vi "喷码内容转换.vi"(10 "输入数据(十进制)":string="123456789") -> (2 "输出数据(十六进制)":string)   [LabVIEW 2020, in "Untitled Library 1.lvlib"]
uses:
  Untitled Library 1.lvlib
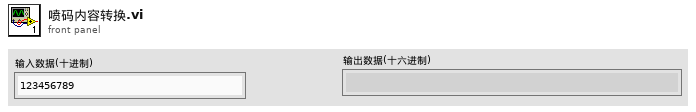
[diagram p1: front panel]
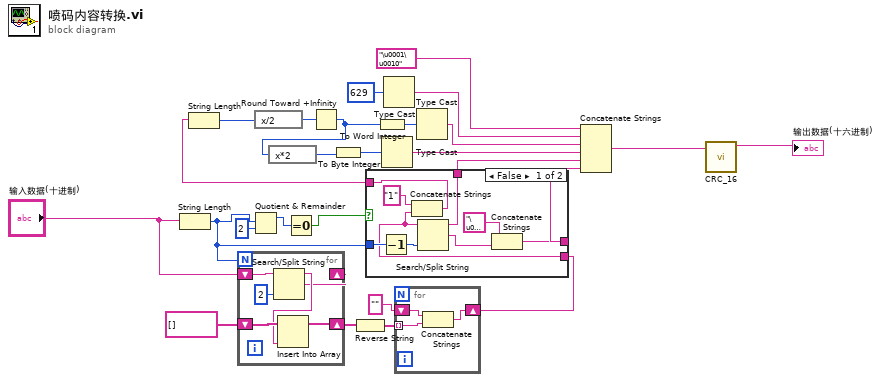
[diagram p0: block diagram]
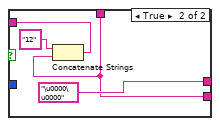
[diagram p2: hidden frame]
diagram:
  n1 = String Length(string="输入数据(十进制)") -> (length=w4:i32)
  n2 = for {
    N: w4 -> [_]
    shift-right: [w31] -> w21
    shift-left: string[] [] -> [w32]
    shift-right: [w27] -> _
    shift-left: "输入数据(十进制)" -> [w30]
    n3 = Search/Split String(string=w30, offset (0)=2 ("长度（剩余）")) -> (substring before match=w28:string, match + rest of string=w27:string)  [unwired: 1 in, 1 out]
    n4 = Insert Into Array(array=w32, new element=w28) -> (w31:string[])  [unwired: 1 in]
  }
  n5 = Quotient & Remainder(x=w4, y=2) -> (x-y*floor(x/y)=w14:i32)  [unwired: 1 out]
  n6 = Equal To 0?(x=w14) -> (x = 0?=w13:bool)
  n7 = Reverse String(1:w21) -> (0:w20:string[])
  n8 = Type Cast(x=i16 629) -> (*(type *) &x=w23:string)  [unwired: 1 in]
  n9 = for {
    tunnel: w20 -> [w33] mode=indexing
    shift-right: [w34] -> w12
    shift-left: "" -> [w35]
    n10 = Concatenate Strings(w35, w33) -> (w34:string)
  }
  n11 = case shown="False" w13 {
    tunnel: [w41 "\u0000\u0000"] -> w6
    tunnel: [w42 w47] -> w7
    tunnel: w12 -> [w37 w47]
    tunnel: w4 -> [w44 _]
    tunnel: [w36 w45] -> w3
    frame False {
      n12 = Decrement(x=w44) -> (x-1=w43:i32)
      n13 = Concatenate Strings("1" ("字符串"), w37) -> (w36:string)
      n14 = Search/Split String(string=w37, offset (0)=w43) -> (substring before match=w42:string, match + rest of string=w39:string)  [unwired: 1 in, 1 out]
      n15 = Concatenate Strings("\u0000", w39) -> (w41:string)
    }
    frame True {
      n16 = Concatenate Strings("12" ("字符串"), w47) -> (w45:string)
    }
  }
  n17 = String Length(string=w3) -> (length=w10:i32)
  n18 = expression code="x/2"(w10) -> (w11:i32)
  n19 = Round Toward +Infinity(x=w11) -> (ceil(x): smallest int >= x=w8:i32)
  n20 = expression code="x*2"(w8) -> (w9:i32)
  n21 = To Byte Integer(number=w9) -> (8bit integer=w24:i8)
  n22 = To Word Integer(number=w8) -> (16bit integer=w17:i16)
  n23 = Type Cast(x=w24) -> (*(type *) &x=w22:string)  [unwired: 1 in]
  n24 = Type Cast(x=w17) -> (*(type *) &x=w16:string)  [unwired: 1 in]
  n25 = Concatenate Strings("\u0001\u0010", w23, w16, w22, w7, w6) -> (w2:string)
  n26 = call "CRC_16.vi"("String"=w2) -> ("String & CRC-16"=→"输出数据(十六进制)":string)  [unwired: 8 in, 2 out]
